vi "calc_consts_build_function.vi"(1 "Corrected Cell Temperature Mean":dbl, 2 "Salinity":dbl, 3 "HCl Concentration":dbl) -> (0 "model description":T1)   [LabVIEW 2010]
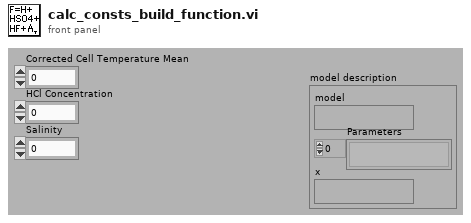
[diagram p1: front panel]
types:
  T1 = cluster{"model":string, "Parameters":string[], "x":string}
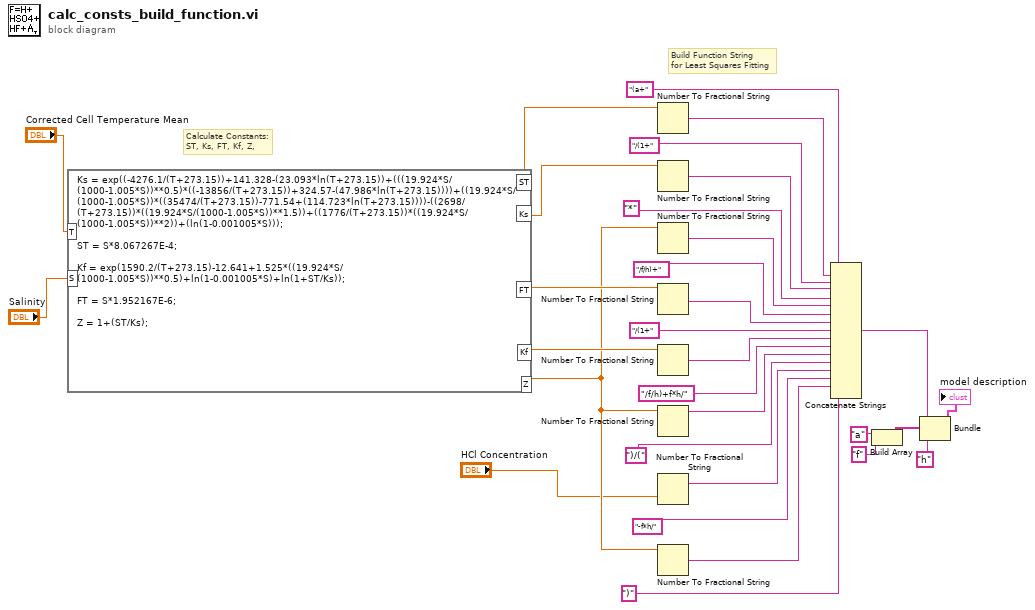
[diagram p0: block diagram]
diagram:
  # "Calculate Constants:\nST, Ks, FT, Kf, Z,"
  # "Build Function String\nfor Least Squares Fitting"
  n1 = formula code="Ks = exp((-4276.1/(T+273.15))+141.328-(23.093*ln(T+273.15))+(((19.924*S/(1000-1.005*S))**0.5)*((-13856/(T+273.15))+324.57-(47.986*ln(T+273.15))))+((19.924*S/(1000-1.005*S))*((35474/(T+273.15))-771.54+(114.723*ln(T+273.15))))-((2698/(T+273.15))*((19.924*S/(1000-1.005*S))**1.5))+((1776/(T+273.15))*((19.924*S/(1000-1.005*S))**2))+(ln(1-0.001005*S)));\n\nST = S*8.067267E-4;\n\nKf = exp(1590.2/(T+273.15)-12.641+1.525*((19.924*S/(1000-1.005*S))**0.5)+ln(1-0.001005*S)+ln(1+ST/Ks));\n\nFT = S*1.952167E-6;\n\nZ = 1+(ST/Ks);"("T"="Corrected Cell Temperature Mean", "S"="Salinity") -> ("Ks"=w27:dbl, "ST"=w26:dbl, "Z"=w28:dbl, "FT"=w29:dbl, "Kf"=w30:dbl)
  n2 = Number To Fractional String(number=w26) -> (F-format string=w10:string)  [unwired: 3 in]
  n3 = Number To Fractional String(number=w27) -> (F-format string=w11:string)  [unwired: 3 in]
  n4 = Number To Fractional String(number=w28) -> (F-format string=w14:string)  [unwired: 3 in]
  n5 = Number To Fractional String(number=w29) -> (F-format string=w16:string)  [unwired: 3 in]
  n6 = Number To Fractional String(number=w30) -> (F-format string=w18:string)  [unwired: 3 in]
  n7 = Number To Fractional String(number=w28) -> (F-format string=w20:string)  [unwired: 3 in]
  n8 = Number To Fractional String(number="HCl Concentration") -> (F-format string=w22:string)  [unwired: 3 in]
  n9 = Number To Fractional String(number=w28) -> (F-format string=w24:string)  [unwired: 3 in]
  n10 = Concatenate Strings("(a+", w10, "/(1+", w11, "*", w14, "/f/h)+", w16, "/(1+", w18, "/f/h)+f*h/", w20, ")/(", w22, "-f*h/", w24, ")") -> (w31:string)
  n11 = Build Array("a", "f") -> (w5:string[])
  n12 = Bundle(w31, w5, "h") -> (→"model description":cluster{string, string[], string})  [unwired: 1 in]
